vi "TagCreatePixelArrayV1Tags.vi"(5 "Layout":string, 6 "Add Border":bool, 7 "Codes":i64[](array[numeric]), 8 "error in (no error)":errorcluster, 11 "ID":i32) -> (0 "error out":errorcluster, 3 "Pixels":u8[][](array[numeric]))   [LabVIEW 2020, in "feature_detection.lvlib"]
uses:
  feature_detection.lvlib
  TagPixelType.ctl
  <vilib>/Utility/error.llb/Error Cluster From Error Code.vi
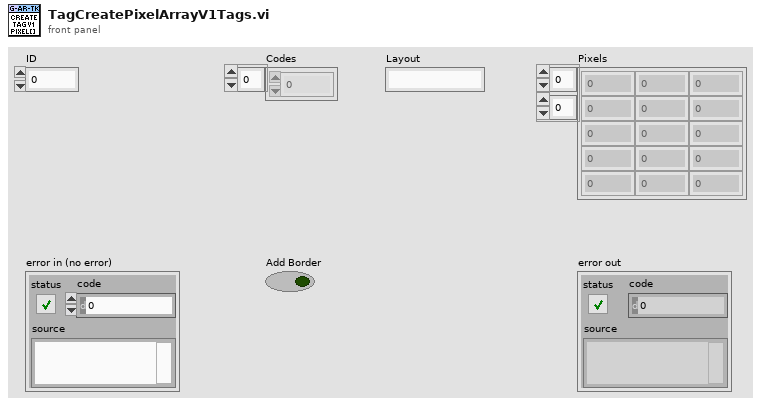
[diagram p1: front panel]
types:
  T1 = typedef "feature_detection.lvlib/TagPixelType.ctl" = enum8{"Black", "White", "Transparent"}
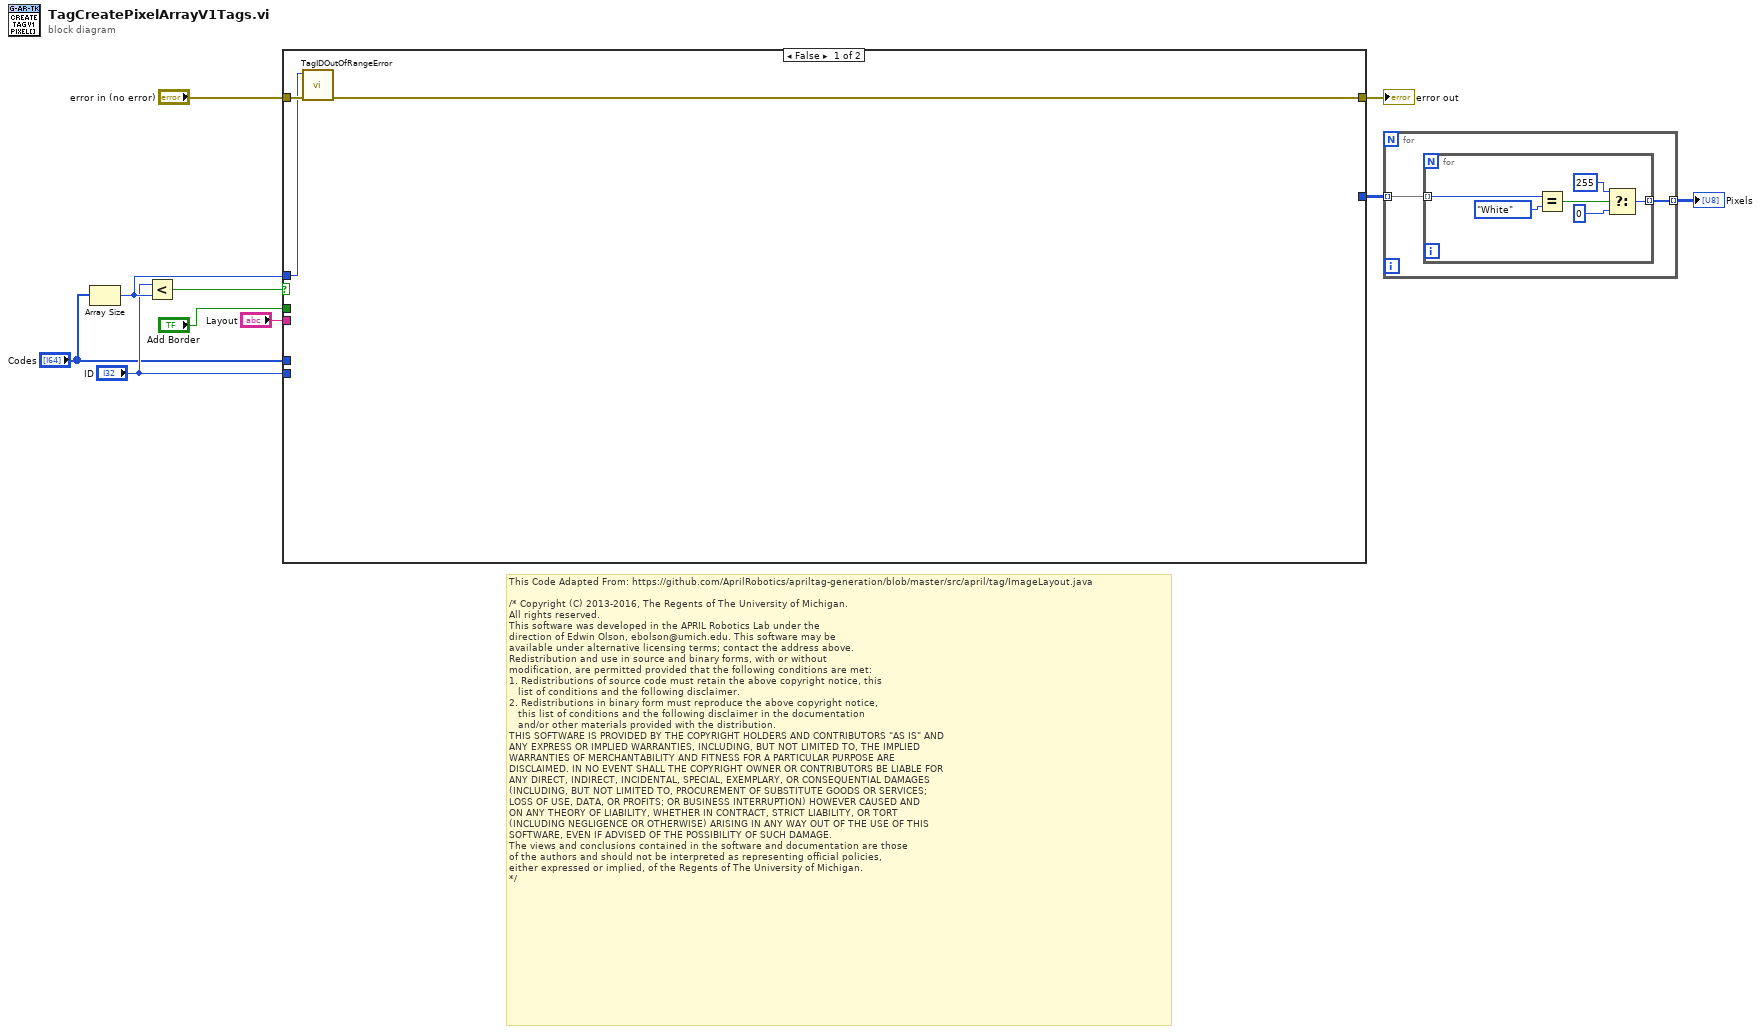
[diagram p0: block diagram]
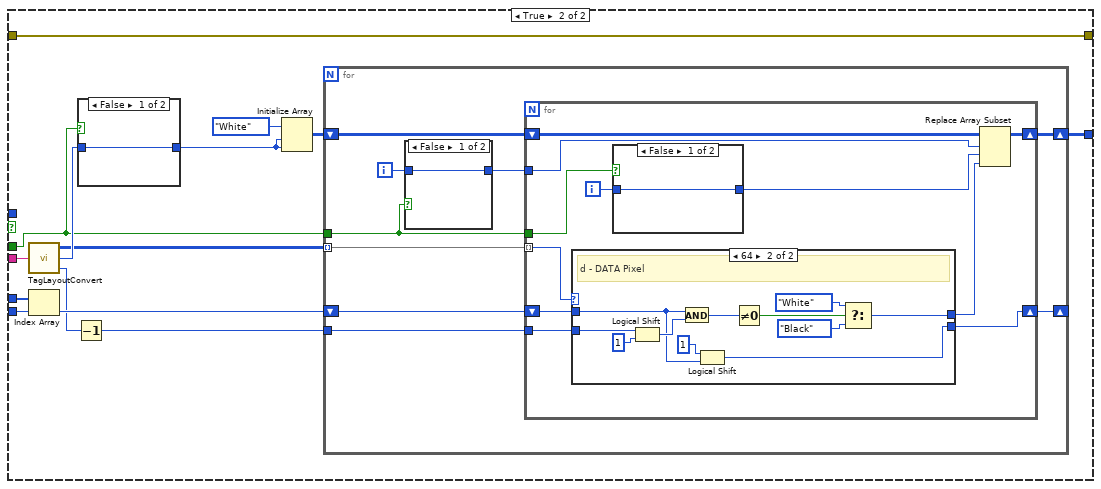
[diagram p2: hidden frame]
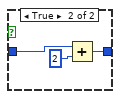
[diagram p3: hidden frame]
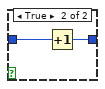
[diagram p4: hidden frame]
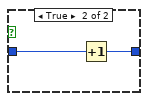
[diagram p5: hidden frame]
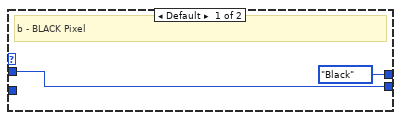
[diagram p6: hidden frame]
diagram:
  # "This Code Adapted From: https://github.com/AprilRobotics/apriltag-generation/blob/master/src/april/tag/ImageLayout.java\n\n/* Copyright (C) 2013-2016, The Regents of The University of Michigan.\nAll rights reserved.\nThis software was developed in the APRIL Robotics Lab under the\ndirection of Edwin Olson, ebolson@umich.edu. This software may be\navailable under alternative licensing terms; contact the address above.\nRedistribution and use in source and binary forms, with or without\nmodification, are permitted provided that the following conditions are met:\n1. Redistributions of source code must retain the above copyright notice, this\n   list of conditions and the following disclaimer.\n2. Redistributions in binary form must reproduce the above copyright notice,\n   this list of conditions and the following disclaimer in the documentation\n   and/or other materials provided with the distribution.\nTHIS SOFTWARE IS PROVIDED BY THE COPYRIGHT HOLDERS AND CONTRIBUTORS \"AS IS\" AND\nANY EXPRESS OR IMPLIED WARRANTIES, INCLUDING, BUT NOT LIMITED TO, THE IMPLIED\nWARRANTIES OF MERCHANTABILITY AND FITNESS FOR A PARTICULAR PURPOSE ARE\nDISCLAIMED. IN NO EVENT SHALL THE COPYRIGHT OWNER OR CONTRIBUTORS BE LIABLE FOR\nANY DIRECT, INDIRECT, INCIDENTAL, SPECIAL, EXEMPLARY, OR CONSEQUENTIAL DAMAGES\n(INCLUDING, BUT NOT LIMITED TO, PROCUREMENT OF SUBSTITUTE GOODS OR SERVICES;\nLOSS OF USE, DATA, OR PROFITS; OR BUSINESS INTERRUPTION) HOWEVER CAUSED AND\nON ANY THEORY OF LIABILITY, WHETHER IN CONTRACT, STRICT LIABILITY, OR TORT\n(INCLUDING NEGLIGENCE OR OTHERWISE) ARISING IN ANY WAY OUT OF THE USE OF THIS\nSOFTWARE, EVEN IF ADVISED OF THE POSSIBILITY OF SUCH DAMAGE.\nThe views and conclusions contained in the software and documentation are those\nof the authors and should not be interpreted as representing official policies,\neither expressed or implied, of the Regents of The University of Michigan.\n*/"
  n1 = Array Size(array="Codes") -> (size(s)=w9:i32)
  n2 = Less?(x="ID", y=w9) -> (x < y?=w6:bool)
  n3 = case shown="False" w6 {
    tunnel: "Codes" -> [_ w27]
    tunnel: "ID" -> [_ w26]
    tunnel: "error in (no error)" -> [w13 w22]
    tunnel: [w12 w22] -> w8
    tunnel: w9 -> [w11 _]
    tunnel: "Layout" -> [_ w24]
    tunnel: [_ w16] -> w3
    tunnel: "Add Border" -> [_ w14]
    frame False {
      n4 = call "TagIDOutOfRangeError.vi"("error in (no error)"=w13, "Tag Family Size"=w11) -> ("error out"=w12:errorcluster)  [unwired: 9 in]
    }
    frame True {
      n5 = call "TagLayoutConvert.vi"("Layout"=w24) -> ("Pixel Map"=w20:u8[][], "Size"=w23:i32, "Number Of Bits"=w18:i32)
      n6 = Index Array(array=w27, index=w26) -> (element=w21:i64)
      n7 = Decrement(x=w18) -> (x-1=w17:i32)
      n8 = case shown="False" w14 {
        tunnel: w23 -> [w28 w31]
        tunnel: [w28 w30] -> w15
        frame False {
        }
        frame True {
          n9 = Add(x=w31, y=2) -> (x+y=w30:i32)
        }
      }
      n10 = Initialize Array(TagPixelType."White", w15, w15) -> (w19:T1[][])
      n11 = for {
        shift-right: [w35] -> _
        shift-left: w21 -> [w36]
        tunnel: w20 -> [w40] mode=indexing
        shift-right: [w34] -> w16
        shift-left: w19 -> [w39]
        tunnel: w17 -> [w37]
        tunnel: w14 -> [w32]
        i -> [w38]
        n12 = case shown="False" w32 {
          tunnel: w38 -> [w41 w43]
          tunnel: [w41 w42] -> w33
          frame False {
          }
          frame True {
            n13 = Increment(x=w43) -> (x+1=w42:i32)
          }
        }
        n14 = for {
          tunnel: w40 -> [w54] mode=indexing
          shift-right: [w52] -> w34
          shift-left: w39 -> [w53]
          tunnel: w33 -> [w50]
          tunnel: w37 -> [w48]
          shift-right: [w46] -> w35
          shift-left: w36 -> [w47]
          tunnel: w32 -> [w44]
          i -> [w49]
          n15 = case shown="64" w54 {
            tunnel: [TagPixelType."Black" ("TagPixelType") w64] -> w51
            tunnel: [w58 w68] -> w46
            tunnel: w48 -> [_ w61]
            tunnel: w47 -> [w58 w60]
            frame Default {
              # "b - BLACK Pixel"
            }
            frame 100 {
              # "d - DATA Pixel"
              n16 = Logical Shift(y=w61, x=i64 1) -> (x << y=w70:i64)
              n17 = And(x=w60, y=w70) -> (x .and. y?=w69:i64)
              n18 = Logical Shift(y=i16 1, x=w60) -> (x << y=w68:i64)
              n19 = Not Equal To 0?(x=w69) -> (x != 0?=w65:bool)
              n20 = Select(t=TagPixelType."White" ("TagPixelType"), s=w65, f=TagPixelType."Black") -> (s? t:f=w64:T1)
            }
          }
          n21 = case shown="False" w44 {
            tunnel: w49 -> [w55 w57]
            tunnel: [w55 w56] -> w45
            frame False {
            }
            frame True {
              n22 = Increment(x=w57) -> (x+1=w56:i32)
            }
          }
          n23 = Replace Array Subset(array=w53, new element=w51, index (row)=w50, index (col)=w45) -> (w52:T1[][])
        }
      }
    }
  }
  "error out" <- w8
  n24 = for {
    tunnel: w3 -> [w72] mode=indexing
    tunnel: [w71] -> w2 mode=indexing
    n25 = for {
      tunnel: w72 -> [w78] mode=indexing
      tunnel: [w74] -> w71 mode=indexing
      n26 = Equal?(x=w78, y=TagPixelType."White") -> (x = y?=w76:bool)
      n27 = Select(t=u8 255, s=w76, f=u8 0) -> (s? t:f=w74:u8)
    }
  }
  "Pixels" <- w2
